vi "S4GUI_002.vi"(7 "Tab ObsEng":enum32{"Obs", "CCD modes", "Eng"}(tab)) -> ()   [LabVIEW 2018] (continued)
                n2402 = call "Next State.vi"("error in (no error)"=w4895, "New_State"=96, "State Machine in"=w4896) -> ("error out"=w4897:errorcluster, "State Machine out"=w4899:refnum<class "State Machine.lvclass">)  [unwired: 7 in]
                n2403 = call-dynamic "Write State Machine.vi"("error in (no error)"=w4897, "State Machine.lvclass"=w4899, "Device in"=w4900) -> ("error out"=w4902:errorcluster, "Device out"=w4903:refnum<class "Channel.lvclass">)  [unwired: 7 in]
                n2404 = call-dynamic "Write Channel.vi"("error in (no error)"=w4902, "Channel.lvclass"=w4903, "Acquisition in"=w4905) -> ("error out"=w4901:errorcluster, "Acquisition out"=w4904:refnum<class "Acquisition.lvclass">)  [unwired: 7 in]
              }
            }
            n2405 = call-dynamic "Write AcquisitionD.vi"("error in (no error)"=w4833, "Acquisition.lvclass"=w4834, "S4ACS_GUI in"=w4837) -> ("error out"=w4877:errorcluster, "S4ACS_GUI out"=w4878:refnum<class "S4GUI.lvclass">)  [unwired: 7 in]
          }
          frame True {
            # "vide S4GUI:\nHandleObservationSync.vi"
            # "aba atual em Tab Acq Type"
            n2406 = call "Read Instrument.lvclass.vi"("error in (no error)"=w4961, "S4ACS_GUI in"=w4962) -> ("error out"=w4964:errorcluster, "Instrument.lvclass"=w4966:refnum<class "Instrument.lvclass">, "S4ACS_GUI out"=w4959:refnum<class "S4GUI.lvclass">)  [unwired: 7 in]
            n2407 = call "Read WPROT.vi"("error in (no error)"=w4964, "Instrument in"=w4966) -> ("error out"=w4963:errorcluster, "Opt_Selector.lvclass"=w4965:refnum<class "Opt_Selector.lvclass">)  [unwired: 7 in, 1 out]
            n2408 = call-dynamic "Read sequencia.vi"("error in (no error)"=w4963, "Opt_Selector in"=w4965) -> ("error out"=w4958:errorcluster, "sequencia"=w4960:u16)  [unwired: 7 in, 1 out]
            n2409 = case shown="\"FOCUS\"" w4952 {
              tunnel: [u32 271 ("Obs_state") u32 251 ("Obs_state")] -> w4986
              tunnel: w4959 -> [w5007 w5010]
              tunnel: w4958 -> [w4997 w5009]
              tunnel: [w5005 w5010] -> w4957
              tunnel: [w4996 w5009] -> w4956
              tunnel: w4955 -> [w5004 _]
              tunnel: w4954 -> [w5003 _]
              tunnel: w4953 -> [w5002 _]
              frame "FOCUS" {
                n2410 = call-dynamic "Read TelFocus.lvclass.vi"("error in (no error)"=w4997, "S4GUI in"=w5007) -> ("error out"=w4999:errorcluster, "TelFocus.lvclass"=w5001:refnum<class "TelFocus.lvclass">, "S4GUI out"=w5006:refnum<class "S4GUI.lvclass">)  [unwired: 7 in]
                n2411 = call-dynamic "LoadParam.vi"("#steps"=w5002, "error in (no error)"=w4999, "step"=w5003, "init"=w5004, "TelFocus in"=w5001) -> ("error out"=w4998:errorcluster, "TelFocus out"=w5000:refnum<class "TelFocus.lvclass">)  [unwired: 5 in]
                n2412 = call-dynamic "Write TelFocus.lvclass.vi"("error in (no error)"=w4998, "TelFocus.lvclass"=w5000, "S4GUI in"=w5006) -> ("error out"=w4996:errorcluster, "S4GUI out"=w5005:refnum<class "S4GUI.lvclass">)  [unwired: 7 in]
              }
              frame Default {
              }
            }
            n2413 = case shown="Default" w4952 {
              tunnel: w4977 -> [_ w4992]
              tunnel: [u32 1 ("# Cycles") w4991] -> w4972
              tunnel: [u32 1 w4990] -> w4967
              tunnel: w4960 -> [_ w4989]
              frame "FOCUS" {
                # "Aba FOCUS: Para a sequencia de foco, sempre  #Cycles=1 e #Seqs=1"
              }
              frame Default {
                n2414 = case shown="True" w4992 {
                  tunnel: [0 w4995] -> w4990
                  tunnel: w4989 -> [_ w4994]
                  frame False {
                    # "OV 20230424: \n#SEQ agora armazena as\nposições da lâmina utilizadas.\nNa fotometria, #SEQ=0"
                    # "fotometria:"
                  }
                  frame True {
                    # "OV 20230424: \n#SEQ agora armazena as\nposições da lâmina utilizadas.\nNa polarimetria, #SEQ=WPROT.sequencia"
                    # "polarimetria:"
                    n2415 = To Unsigned Long Integer(number=w4994) -> (unsigned 32bit integer=w4995:u32)
                  }
                }
                n2416 = local read "# Cycles"() -> (w4991:u32)
              }
            }
            n2417 = call-dynamic "Write Obs_state.vi"("error in (no error)"=w4956, "Obs_state"=w4986, "S4ACS_GUI in"=w4957) -> ("error out"=w4985:errorcluster, "S4ACS_GUI out"=w4984:refnum<class "S4GUI.lvclass">)  [unwired: 7 in]
            n2418 = stacked-sequence {
              seq-local: [w5040 _ _ _] -> [_ w5126 _ _]
              seq-local: [w5039 _ _ _] -> [_ w5125 _ _]
              seq-local: [_ w5124 _ _] -> [_ _ w5187 _]
              seq-local: [_ w5123 _ _] -> [_ _ w5186 _]
              seq-local: [_ _ w5185 _] -> [_ _ _ w5248]
              seq-local: [_ _ w5184 _] -> [_ _ _ w5247]
              tunnel: w4985 -> [w5058 _ _ _]
              tunnel: w4984 -> [w5057 _ _ _]
              tunnel: [_ _ _ w5246] -> w4969
              tunnel: [_ _ _ w5245] -> w4971
              tunnel: w4982 -> [w5038 w5122 w5183 w5244]
              tunnel: w4981 -> [w5037 w5121 w5159 w5220]
              tunnel: w4980 -> [w5036 w5097 w5158 w5219]
              tunnel: w4979 -> [w5035 w5096 w5157 w5218]
              tunnel: w4978 -> [w5030 w5091 w5152 w5213]
              tunnel: w4972 -> [w5027 w5088 w5149 w5210]
              tunnel: w4967 -> [w5022 w5083 w5144 w5205]
              tunnel: w4952 -> [w5016 w5079 w5140 w5199]
              frame #0 {
                # "object"
                # "suffix"
                # "obsType"
                n2419 = local read "Exptime ch1"() -> (w5017:dbl)
                n2420 = call-dynamic "Read AcquisitionA.vi"("error in (no error)"=w5058, "S4ACS_GUI in"=w5057) -> ("error out"=w5056:errorcluster, "Acquisition.lvclass"=w5055:refnum<class "Acquisition.lvclass">, "S4ACS_GUI out"=w5045:refnum<class "S4GUI.lvclass">)  [unwired: 7 in]
                n2421 = call-dynamic "Read Channel.vi"("error in (no error)"=w5056, "Acquisition in"=w5055) -> ("error out"=w5053:errorcluster, "Channel.lvclass"=w5054:refnum<class "Channel.lvclass">, "Acquisition out"=w5044:refnum<class "Acquisition.lvclass">)  [unwired: 7 in]
                n2422 = local read "Exp ch1"() -> (w5042:u32)
                n2423 = call-dynamic "Read Interface.vi"("error in (no error)"=w5053, "Channel in"=w5054) -> ("error out"=w5065:errorcluster, "Interface.lvclass"=w5051:refnum<class "Interface.lvclass">, "Channel out"=w5052:refnum<class "Channel.lvclass">)  [unwired: 7 in]
                n2424 = call "Write Exposure Time.vi"("error in (no error)"=w5065, "Exposure Time"=w5017, "Interface in"=w5051) -> ("error out"=w5018:errorcluster, "Interface out"=w5021:refnum<class "Interface.lvclass">)  [unwired: 7 in]
                n2425 = case shown="Default" w5016 {
                  tunnel: w5021 -> [w5067 w5072]
                  tunnel: [w5067 w5071] -> w5020
                  tunnel: [w5066 w5070] -> w5019
                  tunnel: w5018 -> [w5066 w5069]
                  tunnel: w5017 -> [_ w5068]
                  frame "ZERO" {
                  }
                  frame Default {
                    n2426 = call-dynamic "Write prev ExpTime.vi"("error in (no error)"=w5069, "prev ExpTime"=w5068, "Interface in"=w5072) -> ("error out"=w5070:errorcluster, "Interface out"=w5071:refnum<class "Interface.lvclass">)  [unwired: 7 in]
                  }
                }
                n2427 = call-dynamic "Write Suffix.vi"("error in (no error)"=w5019, "Suffix"=w5038, "Interface in"=w5020) -> ("error out"=w5064:errorcluster, "Interface out"=w5050:refnum<class "Interface.lvclass">)  [unwired: 7 in]
                n2428 = call-dynamic "Write ObsType.vi"("error in (no error)"=w5064, "ObsType"=w5036, "Interface in"=w5050) -> ("error out"=w5063:errorcluster, "Interface out"=w5049:refnum<class "Interface.lvclass">)  [unwired: 7 in]
                n2429 = call-dynamic "Write Object.vi"("error in (no error)"=w5063, "Object"=w5035, "Interface in"=w5049) -> ("error out"=w5062:errorcluster, "Interface out"=w5048:refnum<class "Interface.lvclass">)  [unwired: 7 in]
                n2430 = call-dynamic "Write Comments.vi"("error in (no error)"=w5062, "Comments"=w5037, "Interface in"=w5048) -> ("error out"=w5061:errorcluster, "Interface out"=w5047:refnum<class "Interface.lvclass">)  [unwired: 7 in]
                n2431 = call-dynamic "Write DS9.vi"("error in (no error)"=w5061, "DS9"="F", "Interface in"=w5047) -> ("error out"=w5032:errorcluster, "Interface out"=w5034:refnum<class "Interface.lvclass">)  [unwired: 7 in]
                n2432 = call-dynamic "Write Observer.vi"("error in (no error)"=w5032, "Observer"=w5030, "Interface in"=w5034) -> ("error out"=w5031:errorcluster, "Interface out"=w5033:refnum<class "Interface.lvclass">)  [unwired: 7 in]
                n2433 = call-dynamic "Write # Images.vi"("error in (no error)"=w5031, "# Images"=w5042, "Interface in"=w5033) -> ("error out"=w5059:errorcluster, "Interface out"=w5046:refnum<class "Interface.lvclass">)  [unwired: 7 in]
                n2434 = property on="Exposures Done ch1" class="Slide (strict)"("Scale.Maximum"=w5042, "Scale.Minimum"=0.0 ("Scale.Range:Minimum")) -> ()  [unwired: 2 in, 2 out]
                n2435 = property on="Exposure Time ch1" class="Slide (strict)"("Scale.Maximum"=w5017, "Scale.Minimum"=0.0 ("Scale.Range:Minimum")) -> ()  [unwired: 2 in, 2 out]
                n2436 = call-dynamic "Write Interface.vi"("error in (no error)"=w5059, "Interface.lvclass"=w5046, "Channel in"=w5052) -> ("error out"=w5029:errorcluster, "Channel out"=w5028:refnum<class "Channel.lvclass">)  [unwired: 7 in]
                n2437 = call-dynamic "Write ciclos.vi"("error in (no error)"=w5029, "ciclos"=w5027, "Channel in"=w5028) -> ("error out"=w5024:errorcluster, "Channel out"=w5026:refnum<class "Channel.lvclass">)  [unwired: 7 in]
                n2438 = call-dynamic "Write sequencias.vi"("error in (no error)"=w5024, "sequencias"=w5022, "Channel in"=w5026) -> ("error out"=w5023:errorcluster, "Channel out"=w5025:refnum<class "Channel.lvclass">)  [unwired: 7 in]
                n2439 = call-dynamic "Write Channel.vi"("error in (no error)"=w5023, "Channel.lvclass"=w5025, "Acquisition in"=w5044) -> ("error out"=w5013:errorcluster, "Acquisition out"=w5015:refnum<class "Acquisition.lvclass">)  [unwired: 7 in]
                n2440 = call-dynamic "CalcCubeDuration.vi"("error in (no error)"=w5013, "Acquisition in"=w5015) -> ("error out"=w5012:errorcluster, "Acquisition out"=w5014:refnum<class "Acquisition.lvclass">)  [unwired: 8 in]
                n2441 = call-dynamic "Write AcquisitionA.vi"("error in (no error)"=w5012, "Acquisition.lvclass"=w5014, "S4ACS_GUI in"=w5045) -> ("error out"=w5039:errorcluster, "S4ACS_GUI out"=w5040:refnum<class "S4GUI.lvclass">)  [unwired: 7 in]
              }
              frame #1 {
                # "object"
                # "suffix"
                # "obsType"
                n2442 = call "Read AcquisitionB.vi"("error in (no error)"=w5125, "S4ACS_GUI in"=w5126) -> ("error out"=w5108:errorcluster, "Acquisition.lvclass"=w5109:refnum<class "Acquisition.lvclass">, "S4ACS_GUI out"=w5119:refnum<class "S4GUI.lvclass">)  [unwired: 7 in]
                n2443 = local read "Exptime ch2"() -> (w5080:dbl)
                n2444 = call-dynamic "Read Channel.vi"("error in (no error)"=w5108, "Acquisition in"=w5109) -> ("error out"=w5111:errorcluster, "Channel.lvclass"=w5110:refnum<class "Channel.lvclass">, "Acquisition out"=w5120:refnum<class "Acquisition.lvclass">)  [unwired: 7 in]
                n2445 = call-dynamic "Read Interface.vi"("error in (no error)"=w5111, "Channel in"=w5110) -> ("error out"=w5102:errorcluster, "Interface.lvclass"=w5113:refnum<class "Interface.lvclass">, "Channel out"=w5112:refnum<class "Channel.lvclass">)  [unwired: 7 in]
                n2446 = call "Write Exposure Time.vi"("error in (no error)"=w5102, "Exposure Time"=w5080, "Interface in"=w5113) -> ("error out"=w5081:errorcluster, "Interface out"=w5082:refnum<class "Interface.lvclass">)  [unwired: 7 in]
                n2447 = case shown="Default" w5079 {
                  tunnel: w5082 -> [w5128 w5133]
                  tunnel: [w5128 w5132] -> w5078
                  tunnel: [w5127 w5131] -> w5077
                  tunnel: w5081 -> [w5127 w5130]
                  tunnel: w5080 -> [_ w5129]
                  frame "ZERO" {
                  }
                  frame Default {
                    n2448 = call-dynamic "Write prev ExpTime.vi"("error in (no error)"=w5130, "prev ExpTime"=w5129, "Interface in"=w5133) -> ("error out"=w5131:errorcluster, "Interface out"=w5132:refnum<class "Interface.lvclass">)  [unwired: 7 in]
                  }
                }
                n2449 = call-dynamic "Write Suffix.vi"("error in (no error)"=w5077, "Suffix"=w5122, "Interface in"=w5078) -> ("error out"=w5103:errorcluster, "Interface out"=w5114:refnum<class "Interface.lvclass">)  [unwired: 7 in]
                n2450 = call-dynamic "Write ObsType.vi"("error in (no error)"=w5103, "ObsType"=w5097, "Interface in"=w5114) -> ("error out"=w5104:errorcluster, "Interface out"=w5115:refnum<class "Interface.lvclass">)  [unwired: 7 in]
                n2451 = call-dynamic "Write Object.vi"("error in (no error)"=w5104, "Object"=w5096, "Interface in"=w5115) -> ("error out"=w5105:errorcluster, "Interface out"=w5116:refnum<class "Interface.lvclass">)  [unwired: 7 in]
                n2452 = call-dynamic "Write Comments.vi"("error in (no error)"=w5105, "Comments"=w5121, "Interface in"=w5116) -> ("error out"=w5106:errorcluster, "Interface out"=w5117:refnum<class "Interface.lvclass">)  [unwired: 7 in]
                n2453 = local read "Exp ch2"() -> (w5100:u32)
                n2454 = call-dynamic "Write DS9.vi"("error in (no error)"=w5106, "DS9"="F", "Interface in"=w5117) -> ("error out"=w5093:errorcluster, "Interface out"=w5095:refnum<class "Interface.lvclass">)  [unwired: 7 in]
                n2455 = call-dynamic "Write Observer.vi"("error in (no error)"=w5093, "Observer"=w5091, "Interface in"=w5095) -> ("error out"=w5092:errorcluster, "Interface out"=w5094:refnum<class "Interface.lvclass">)  [unwired: 7 in]
                n2456 = call-dynamic "Write # Images.vi"("error in (no error)"=w5092, "# Images"=w5100, "Interface in"=w5094) -> ("error out"=w5107:errorcluster, "Interface out"=w5118:refnum<class "Interface.lvclass">)  [unwired: 7 in]
                n2457 = property on="Exposure Time ch2" class="Slide (strict)"("Scale.Maximum"=w5080, "Scale.Minimum"=0.0 ("Scale.Range:Minimum")) -> ()  [unwired: 2 in, 2 out]
                n2458 = property on="Exposures Done ch2" class="Slide (strict)"("Scale.Maximum"=w5100, "Scale.Minimum"=0.0 ("Scale.Range:Minimum")) -> ()  [unwired: 2 in, 2 out]
                n2459 = call-dynamic "Write Interface.vi"("error in (no error)"=w5107, "Interface.lvclass"=w5118, "Channel in"=w5112) -> ("error out"=w5090:errorcluster, "Channel out"=w5089:refnum<class "Channel.lvclass">)  [unwired: 7 in]
                n2460 = call-dynamic "Write ciclos.vi"("error in (no error)"=w5090, "ciclos"=w5088, "Channel in"=w5089) -> ("error out"=w5085:errorcluster, "Channel out"=w5087:refnum<class "Channel.lvclass">)  [unwired: 7 in]
                n2461 = call-dynamic "Write sequencias.vi"("error in (no error)"=w5085, "sequencias"=w5083, "Channel in"=w5087) -> ("error out"=w5084:errorcluster, "Channel out"=w5086:refnum<class "Channel.lvclass">)  [unwired: 7 in]
                n2462 = call-dynamic "Write Channel.vi"("error in (no error)"=w5084, "Channel.lvclass"=w5086, "Acquisition in"=w5120) -> ("error out"=w5074:errorcluster, "Acquisition out"=w5076:refnum<class "Acquisition.lvclass">)  [unwired: 7 in]
                n2463 = call-dynamic "CalcCubeDuration.vi"("error in (no error)"=w5074, "Acquisition in"=w5076) -> ("error out"=w5073:errorcluster, "Acquisition out"=w5075:refnum<class "Acquisition.lvclass">)  [unwired: 8 in]
                n2464 = call "Write AcquisitionB.vi"("error in (no error)"=w5073, "Acquisition.lvclass"=w5075, "S4ACS_GUI in"=w5119) -> ("error out"=w5123:errorcluster, "S4ACS_GUI out"=w5124:refnum<class "S4GUI.lvclass">)  [unwired: 7 in]
              }
              frame #2 {
                # "object"
                # "suffix"
                # "obsType"
                n2465 = call-dynamic "Read AcquisitionC.vi"("error in (no error)"=w5186, "S4ACS_GUI in"=w5187) -> ("error out"=w5176:errorcluster, "Acquisition.lvclass"=w5175:refnum<class "Acquisition.lvclass">, "S4ACS_GUI out"=w5165:refnum<class "S4GUI.lvclass">)  [unwired: 7 in]
                n2466 = call-dynamic "Read Channel.vi"("error in (no error)"=w5176, "Acquisition in"=w5175) -> ("error out"=w5173:errorcluster, "Channel.lvclass"=w5174:refnum<class "Channel.lvclass">, "Acquisition out"=w5164:refnum<class "Acquisition.lvclass">)  [unwired: 7 in]
                n2467 = local read "Exptime ch3"() -> (w5141:dbl)
                n2468 = call-dynamic "Read Interface.vi"("error in (no error)"=w5173, "Channel in"=w5174) -> ("error out"=w5182:errorcluster, "Interface.lvclass"=w5171:refnum<class "Interface.lvclass">, "Channel out"=w5172:refnum<class "Channel.lvclass">)  [unwired: 7 in]
                n2469 = call "Write Exposure Time.vi"("error in (no error)"=w5182, "Exposure Time"=w5141, "Interface in"=w5171) -> ("error out"=w5142:errorcluster, "Interface out"=w5143:refnum<class "Interface.lvclass">)  [unwired: 7 in]
                n2470 = case shown="\"ZERO\"" w5140 {
                  tunnel: w5143 -> [w5189 w5194]
                  tunnel: [w5189 w5193] -> w5139
                  tunnel: [w5188 w5192] -> w5138
                  tunnel: w5142 -> [w5188 w5191]
                  tunnel: w5141 -> [_ w5190]
                  frame "ZERO" {
                  }
                  frame Default {
                    n2471 = call-dynamic "Write prev ExpTime.vi"("error in (no error)"=w5191, "prev ExpTime"=w5190, "Interface in"=w5194) -> ("error out"=w5192:errorcluster, "Interface out"=w5193:refnum<class "Interface.lvclass">)  [unwired: 7 in]
                  }
                }
                n2472 = call-dynamic "Write Suffix.vi"("error in (no error)"=w5138, "Suffix"=w5183, "Interface in"=w5139) -> ("error out"=w5181:errorcluster, "Interface out"=w5170:refnum<class "Interface.lvclass">)  [unwired: 7 in]
                n2473 = call-dynamic "Write ObsType.vi"("error in (no error)"=w5181, "ObsType"=w5158, "Interface in"=w5170) -> ("error out"=w5180:errorcluster, "Interface out"=w5169:refnum<class "Interface.lvclass">)  [unwired: 7 in]
                n2474 = call-dynamic "Write Object.vi"("error in (no error)"=w5180, "Object"=w5157, "Interface in"=w5169) -> ("error out"=w5179:errorcluster, "Interface out"=w5168:refnum<class "Interface.lvclass">)  [unwired: 7 in]
                n2475 = call-dynamic "Write Comments.vi"("error in (no error)"=w5179, "Comments"=w5159, "Interface in"=w5168) -> ("error out"=w5178:errorcluster, "Interface out"=w5167:refnum<class "Interface.lvclass">)  [unwired: 7 in]
                n2476 = call-dynamic "Write DS9.vi"("error in (no error)"=w5178, "DS9"="F", "Interface in"=w5167) -> ("error out"=w5154:errorcluster, "Interface out"=w5156:refnum<class "Interface.lvclass">)  [unwired: 7 in]
                n2477 = local read "Exp ch3"() -> (w5162:u32)
                n2478 = property on="Exposure Time ch3" class="Slide (strict)"("Scale.Maximum"=w5141, "Scale.Minimum"=0.0 ("Scale.Range:Minimum")) -> ()  [unwired: 2 in, 2 out]
                n2479 = call-dynamic "Write Observer.vi"("error in (no error)"=w5154, "Observer"=w5152, "Interface in"=w5156) -> ("error out"=w5153:errorcluster, "Interface out"=w5155:refnum<class "Interface.lvclass">)  [unwired: 7 in]
                n2480 = property on="Exposures Done ch3" class="Slide (strict)"("Scale.Maximum"=w5162, "Scale.Minimum"=0.0 ("Scale.Range:Minimum")) -> ()  [unwired: 2 in, 2 out]
                n2481 = call-dynamic "Write # Images.vi"("error in (no error)"=w5153, "# Images"=w5162, "Interface in"=w5155) -> ("error out"=w5177:errorcluster, "Interface out"=w5166:refnum<class "Interface.lvclass">)  [unwired: 7 in]
                n2482 = call-dynamic "Write Interface.vi"("error in (no error)"=w5177, "Interface.lvclass"=w5166, "Channel in"=w5172) -> ("error out"=w5151:errorcluster, "Channel out"=w5150:refnum<class "Channel.lvclass">)  [unwired: 7 in]
                n2483 = call-dynamic "Write ciclos.vi"("error in (no error)"=w5151, "ciclos"=w5149, "Channel in"=w5150) -> ("error out"=w5146:errorcluster, "Channel out"=w5148:refnum<class "Channel.lvclass">)  [unwired: 7 in]
                n2484 = call-dynamic "Write sequencias.vi"("error in (no error)"=w5146, "sequencias"=w5144, "Channel in"=w5148) -> ("error out"=w5145:errorcluster, "Channel out"=w5147:refnum<class "Channel.lvclass">)  [unwired: 7 in]
                n2485 = call-dynamic "Write Channel.vi"("error in (no error)"=w5145, "Channel.lvclass"=w5147, "Acquisition in"=w5164) -> ("error out"=w5135:errorcluster, "Acquisition out"=w5137:refnum<class "Acquisition.lvclass">)  [unwired: 7 in]
                n2486 = call-dynamic "CalcCubeDuration.vi"("error in (no error)"=w5135, "Acquisition in"=w5137) -> ("error out"=w5134:errorcluster, "Acquisition out"=w5136:refnum<class "Acquisition.lvclass">)  [unwired: 8 in]
                n2487 = call-dynamic "Write AcquisitionC.vi"("error in (no error)"=w5134, "Acquisition.lvclass"=w5136, "S4ACS_GUI in"=w5165) -> ("error out"=w5184:errorcluster, "S4ACS_GUI out"=w5185:refnum<class "S4GUI.lvclass">)  [unwired: 7 in]
              }
              frame #3 {
                # "object"
                # "suffix"
                # "obsType"
                n2488 = call-dynamic "Read AcquisitionD.vi"("error in (no error)"=w5247, "S4ACS_GUI in"=w5248) -> ("error out"=w5237:errorcluster, "Acquisition.lvclass"=w5236:refnum<class "Acquisition.lvclass">, "S4ACS_GUI out"=w5226:refnum<class "S4GUI.lvclass">)  [unwired: 7 in]
                n2489 = local read "Exptime ch4"() -> (w5200:dbl)
                n2490 = call-dynamic "Read Channel.vi"("error in (no error)"=w5237, "Acquisition in"=w5236) -> ("error out"=w5234:errorcluster, "Channel.lvclass"=w5235:refnum<class "Channel.lvclass">, "Acquisition out"=w5225:refnum<class "Acquisition.lvclass">)  [unwired: 7 in]
                n2491 = call-dynamic "Read Interface.vi"("error in (no error)"=w5234, "Channel in"=w5235) -> ("error out"=w5243:errorcluster, "Interface.lvclass"=w5232:refnum<class "Interface.lvclass">, "Channel out"=w5233:refnum<class "Channel.lvclass">)  [unwired: 7 in]
                n2492 = call "Write Exposure Time.vi"("error in (no error)"=w5243, "Exposure Time"=w5200, "Interface in"=w5232) -> ("error out"=w5202:errorcluster, "Interface out"=w5204:refnum<class "Interface.lvclass">)  [unwired: 7 in]
                n2493 = case shown="Default" w5199 {
                  tunnel: w5204 -> [w5250 w5255]
                  tunnel: [w5250 w5254] -> w5203
                  tunnel: [w5249 w5253] -> w5201
                  tunnel: w5202 -> [w5249 w5252]
                  tunnel: w5200 -> [_ w5251]
                  frame "ZERO" {
                  }
                  frame Default {
                    n2494 = call-dynamic "Write prev ExpTime.vi"("error in (no error)"=w5252, "prev ExpTime"=w5251, "Interface in"=w5255) -> ("error out"=w5253:errorcluster, "Interface out"=w5254:refnum<class "Interface.lvclass">)  [unwired: 7 in]
                  }
                }
                n2495 = call-dynamic "Write Suffix.vi"("error in (no error)"=w5201, "Suffix"=w5244, "Interface in"=w5203) -> ("error out"=w5242:errorcluster, "Interface out"=w5231:refnum<class "Interface.lvclass">)  [unwired: 7 in]
                n2496 = call-dynamic "Write ObsType.vi"("error in (no error)"=w5242, "ObsType"=w5219, "Interface in"=w5231) -> ("error out"=w5241:errorcluster, "Interface out"=w5230:refnum<class "Interface.lvclass">)  [unwired: 7 in]
                n2497 = call-dynamic "Write Object.vi"("error in (no error)"=w5241, "Object"=w5218, "Interface in"=w5230) -> ("error out"=w5240:errorcluster, "Interface out"=w5229:refnum<class "Interface.lvclass">)  [unwired: 7 in]
                n2498 = call-dynamic "Write Comments.vi"("error in (no error)"=w5240, "Comments"=w5220, "Interface in"=w5229) -> ("error out"=w5239:errorcluster, "Interface out"=w5228:refnum<class "Interface.lvclass">)  [unwired: 7 in]
                n2499 = call-dynamic "Write DS9.vi"("error in (no error)"=w5239, "DS9"="F", "Interface in"=w5228) -> ("error out"=w5215:errorcluster, "Interface out"=w5217:refnum<class "Interface.lvclass">)  [unwired: 7 in]
                n2500 = property on="Exposure Time ch4" class="Slide (strict)"("Scale.Maximum"=w5200, "Scale.Minimum"=0.0 ("Scale.Range:Minimum")) -> ()  [unwired: 2 in, 2 out]
                n2501 = local read "Exp ch4"() -> (w5223:u32)
                n2502 = call-dynamic "Write Observer.vi"("error in (no error)"=w5215, "Observer"=w5213, "Interface in"=w5217) -> ("error out"=w5214:errorcluster, "Interface out"=w5216:refnum<class "Interface.lvclass">)  [unwired: 7 in]
                n2503 = property on="Exposures Done ch4" class="Slide (strict)"("Scale.Maximum"=w5223, "Scale.Minimum"=0.0 ("Scale.Range:Minimum")) -> ()  [unwired: 2 in, 2 out]
                n2504 = call-dynamic "Write # Images.vi"("error in (no error)"=w5214, "# Images"=w5223, "Interface in"=w5216) -> ("error out"=w5238:errorcluster, "Interface out"=w5227:refnum<class "Interface.lvclass">)  [unwired: 7 in]
                n2505 = call-dynamic "Write Interface.vi"("error in (no error)"=w5238, "Interface.lvclass"=w5227, "Channel in"=w5233) -> ("error out"=w5212:errorcluster, "Channel out"=w5211:refnum<class "Channel.lvclass">)  [unwired: 7 in]
                n2506 = call-dynamic "Write ciclos.vi"("error in (no error)"=w5212, "ciclos"=w5210, "Channel in"=w5211) -> ("error out"=w5208:errorcluster, "Channel out"=w5209:refnum<class "Channel.lvclass">)  [unwired: 7 in]
                n2507 = call-dynamic "Write sequencias.vi"("error in (no error)"=w5208, "sequencias"=w5205, "Channel in"=w5209) -> ("error out"=w5207:errorcluster, "Channel out"=w5206:refnum<class "Channel.lvclass">)  [unwired: 7 in]
                n2508 = call-dynamic "Write Channel.vi"("error in (no error)"=w5207, "Channel.lvclass"=w5206, "Acquisition in"=w5225) -> ("error out"=w5196:errorcluster, "Acquisition out"=w5198:refnum<class "Acquisition.lvclass">)  [unwired: 7 in]
                n2509 = call-dynamic "CalcCubeDuration.vi"("error in (no error)"=w5196, "Acquisition in"=w5198) -> ("error out"=w5195:errorcluster, "Acquisition out"=w5197:refnum<class "Acquisition.lvclass">)  [unwired: 8 in]
                n2510 = call-dynamic "Write AcquisitionD.vi"("error in (no error)"=w5195, "Acquisition.lvclass"=w5197, "S4ACS_GUI in"=w5226) -> ("error out"=w5245:errorcluster, "S4ACS_GUI out"=w5246:refnum<class "S4GUI.lvclass">)  [unwired: 7 in]
              }
            }
            n2511 = call-dynamic "Write sequencias.vi"("error in (no error)"=w4971, "sequencias"=w4967, "S4GUI in"=w4969) -> ("error out"=w4970:errorcluster, "S4GUI out"=w4968:refnum<class "S4GUI.lvclass">)  [unwired: 7 in]
            n2512 = call-dynamic "Write ciclos.vi"("error in (no error)"=w4970, "ciclos"=w4972, "S4ACS_GUI in"=w4968) -> ("error out"=w4974:errorcluster, "S4ACS_GUI out"=w4976:refnum<class "S4GUI.lvclass">)  [unwired: 7 in]
            n2513 = property on="#Cycles Done" class="Slide (strict)"("Scale.Maximum"=w4972, "Scale.Minimum"=0.0 ("Scale.Range:Minor Increment")) -> ()  [unwired: 2 in, 2 out]
            n2514 = call-dynamic "Write TotalCiclos.vi"("error in (no error)"=w4974, "TotalCiclos"=w4972, "S4GUI in"=w4976) -> ("error out"=w4973:errorcluster, "S4GUI out"=w4975:refnum<class "S4GUI.lvclass">)  [unwired: 7 in]
          }
        }
        n2515 = call-dynamic "Write User Event.vi"("error in (no error)"=w4808, "User Event"=w4805, "S4GUI in"=w4809) -> ("error out"=w4807:errorcluster, "S4GUI out"=w4806:refnum<class "S4GUI.lvclass">)  [unwired: 7 in]
        n2516 = property on="Pause SM" class="Bool"(error in=w4807, "DisabledEnum"=T12."Enabled" ("Disabled")) -> (error out=w4826:errorcluster)  [unwired: 1 in, 1 out]
      }
      event "# Cycles": Value Change {
        w5256 = 0.0 ("Scale.Range:Minor Increment")
        n2517 = event-data() -> ("NewVal"=w5257:u32)  [unwired: 1 in]
        n2518 = call-dynamic "Write ciclos.vi"("error in (no error)"=w5260, "ciclos"=w5257, "S4ACS_GUI in"=w5261) -> ("error out"=w5259:errorcluster, "S4ACS_GUI out"=w5258:refnum<class "S4GUI.lvclass">)  [unwired: 7 in]
        n2519 = property on="#Cycles Done" class="Slide (strict)"("Scale.Maximum"=w5257, "Scale.Minimum"=w5256) -> ()  [unwired: 2 in, 2 out]
        n2520 = property on="Cycles Done ch2" class="Slide (strict)"("Scale.Maximum"=w5257, "Scale.Minimum"=w5256) -> ()  [unwired: 2 in, 2 out]
        n2521 = property on="Cycles Done ch4" class="Slide (strict)"("Scale.Maximum"=w5257, "Scale.Minimum"=w5256) -> ()  [unwired: 2 in, 2 out]
        n2522 = property on="Cycles Done ch1" class="Slide (strict)"("Scale.Maximum"=w5257, "Scale.Minimum"=w5256) -> ()  [unwired: 2 in, 2 out]
        n2523 = property on="Cycles Done ch3" class="Slide (strict)"("Scale.Maximum"=w5257, "Scale.Minimum"=w5256) -> ()  [unwired: 2 in, 2 out]
      }
      event "AllConfig": Value Change {
        n2524 = event-data() -> ()  [unwired: 1 in, 6 out]
        n2525 = call "Read Instrument.lvclass.vi"("error in (no error)"=w5266, "S4ACS_GUI in"=w5267) -> ("error out"=w5346:errorcluster, "Instrument.lvclass"=w5313:refnum<class "Instrument.lvclass">, "S4ACS_GUI out"=w5344:refnum<class "S4GUI.lvclass">)  [unwired: 7 in]
        n2526 = call "Read ASEL.vi"("error in (no error)"=w5346, "Instrument in"=w5313) -> ("error out"=w5338:errorcluster, "Opt_Selector.lvclass"=w5337:refnum<class "Opt_Selector.lvclass">, "Instrument out"=w5345:refnum<class "Instrument.lvclass">)  [unwired: 7 in]
        n2527 = call-dynamic "Read State Machine.vi"("error in (no error)"=w5338, "Device in"=w5337) -> ("error out"=w5341:errorcluster, "State Machine.lvclass"=w5343:refnum<class "State Machine.lvclass">, "Device out"=w5335:refnum<class "Opt_Selector.lvclass">)  [unwired: 7 in]
        n2528 = call "Next State.vi"("error in (no error)"=w5341, "New_State"=1, "State Machine in"=w5343) -> ("error out"=w5340:errorcluster, "State Machine out"=w5339:refnum<class "State Machine.lvclass">)  [unwired: 7 in]
        n2529 = call-dynamic "Write State Machine.vi"("error in (no error)"=w5340, "State Machine.lvclass"=w5339, "Device in"=w5335) -> ("error out"=w5334:errorcluster, "Device out"=w5336:refnum<class "Opt_Selector.lvclass">)  [unwired: 7 in]
        n2530 = call "Write ASEL.vi"("error in (no error)"=w5334, "Opt_Selector.lvclass"=w5336, "Instrument in"=w5345) -> ("error out"=w5296:errorcluster, "Instrument out"=w5312:refnum<class "Instrument.lvclass">)  [unwired: 7 in]
        n2531 = call "Read CALW.vi"("error in (no error)"=w5296, "Instrument in"=w5312) -> ("error out"=w5329:errorcluster, "Opt_Selector.lvclass"=w5330:refnum<class "Opt_Selector.lvclass">, "Instrument out"=w5311:refnum<class "Instrument.lvclass">)  [unwired: 7 in]
        n2532 = call-dynamic "Read State Machine.vi"("error in (no error)"=w5329, "Device in"=w5330) -> ("error out"=w5326:errorcluster, "State Machine.lvclass"=w5324:refnum<class "State Machine.lvclass">, "Device out"=w5332:refnum<class "Opt_Selector.lvclass">)  [unwired: 7 in]
        n2533 = call "Next State.vi"("error in (no error)"=w5326, "New_State"=1, "State Machine in"=w5324) -> ("error out"=w5327:errorcluster, "State Machine out"=w5328:refnum<class "State Machine.lvclass">)  [unwired: 7 in]
        n2534 = call-dynamic "Write State Machine.vi"("error in (no error)"=w5327, "State Machine.lvclass"=w5328, "Device in"=w5332) -> ("error out"=w5333:errorcluster, "Device out"=w5331:refnum<class "Opt_Selector.lvclass">)  [unwired: 7 in]
        n2535 = call "Write CALW.vi"("error in (no error)"=w5333, "Opt_Selector.lvclass"=w5331, "Instrument in"=w5311) -> ("error out"=w5295:errorcluster, "Instrument out"=w5310:refnum<class "Instrument.lvclass">)  [unwired: 7 in]
        n2536 = call "Read WPSEL.vi"("error in (no error)"=w5295, "Instrument in"=w5310) -> ("error out"=w5318:errorcluster, "Opt_Selector.lvclass"=w5317:refnum<class "Opt_Selector.lvclass">, "Instrument out"=w5309:refnum<class "Instrument.lvclass">)  [unwired: 7 in]
        n2537 = call-dynamic "Read State Machine.vi"("error in (no error)"=w5318, "Device in"=w5317) -> ("error out"=w5321:errorcluster, "State Machine.lvclass"=w5323:refnum<class "State Machine.lvclass">, "Device out"=w5315:refnum<class "Opt_Selector.lvclass">)  [unwired: 7 in]
        n2538 = call "Next State.vi"("error in (no error)"=w5321, "New_State"=1, "State Machine in"=w5323) -> ("error out"=w5320:errorcluster, "State Machine out"=w5319:refnum<class "State Machine.lvclass">)  [unwired: 7 in]
        n2539 = call-dynamic "Write State Machine.vi"("error in (no error)"=w5320, "State Machine.lvclass"=w5319, "Device in"=w5315) -> ("error out"=w5314:errorcluster, "Device out"=w5316:refnum<class "Opt_Selector.lvclass">)  [unwired: 7 in]
        n2540 = call "Write WPSEL.vi"("error in (no error)"=w5314, "Opt_Selector.lvclass"=w5316, "Instrument in"=w5309) -> ("error out"=w5294:errorcluster, "Instrument out"=w5298:refnum<class "Instrument.lvclass">)  [unwired: 7 in]
        n2541 = call "Read WPROT.vi"("error in (no error)"=w5294, "Instrument in"=w5298) -> ("error out"=w5304:errorcluster, "Opt_Selector.lvclass"=w5305:refnum<class "Opt_Selector.lvclass">, "Instrument out"=w5297:refnum<class "Instrument.lvclass">)  [unwired: 7 in]
        n2542 = call-dynamic "Read State Machine.vi"("error in (no error)"=w5304, "Device in"=w5305) -> ("error out"=w5301:errorcluster, "State Machine.lvclass"=w5299:refnum<class "State Machine.lvclass">, "Device out"=w5307:refnum<class "Opt_Selector.lvclass">)  [unwired: 7 in]
        n2543 = call "Next State.vi"("error in (no error)"=w5301, "New_State"=1, "State Machine in"=w5299) -> ("error out"=w5302:errorcluster, "State Machine out"=w5303:refnum<class "State Machine.lvclass">)  [unwired: 7 in]
        n2544 = call-dynamic "Write State Machine.vi"("error in (no error)"=w5302, "State Machine.lvclass"=w5303, "Device in"=w5307) -> ("error out"=w5308:errorcluster, "Device out"=w5306:refnum<class "Opt_Selector.lvclass">)  [unwired: 7 in]
        n2545 = call "Write WPROT.vi"("error in (no error)"=w5308, "Opt_Selector.lvclass"=w5306, "Instrument in"=w5297) -> ("error out"=w5270:errorcluster, "Instrument out"=w5271:refnum<class "Instrument.lvclass">)  [unwired: 7 in]
        n2546 = call "Read GMIR.vi"("error in (no error)"=w5270, "Instrument in"=w5271) -> ("error out"=w5289:errorcluster, "Opt_Continuous.lvclass"=w5290:refnum<class "Opt_Continuous.lvclass">, "Instrument out"=w5283:refnum<class "Instrument.lvclass">)  [unwired: 7 in]
        n2547 = call-dynamic "Read State Machine.vi"("error in (no error)"=w5289, "Device in"=w5290) -> ("error out"=w5286:errorcluster, "State Machine.lvclass"=w5284:refnum<class "State Machine.lvclass">, "Device out"=w5292:refnum<class "Opt_Continuous.lvclass">)  [unwired: 7 in]
        n2548 = call "Next State.vi"("error in (no error)"=w5286, "New_State"=1, "State Machine in"=w5284) -> ("error out"=w5287:errorcluster, "State Machine out"=w5288:refnum<class "State Machine.lvclass">)  [unwired: 7 in]
        n2549 = call-dynamic "Write State Machine.vi"("error in (no error)"=w5287, "State Machine.lvclass"=w5288, "Device in"=w5292) -> ("error out"=w5293:errorcluster, "Device out"=w5291:refnum<class "Opt_Continuous.lvclass">)  [unwired: 7 in]
        n2550 = call "Write GMIR.vi"("error in (no error)"=w5293, "Opt_Continuous.lvclass"=w5291, "Instrument in"=w5283) -> ("error out"=w5268:errorcluster, "Instrument out"=w5269:refnum<class "Instrument.lvclass">)  [unwired: 7 in]
        n2551 = call "Read GFOC.vi"("error in (no error)"=w5268, "Instrument in"=w5269) -> ("error out"=w5278:errorcluster, "Opt_Continuous.lvclass"=w5279:refnum<class "Opt_Continuous.lvclass">, "Instrument out"=w5272:refnum<class "Instrument.lvclass">)  [unwired: 7 in]
        n2552 = call-dynamic "Read State Machine.vi"("error in (no error)"=w5278, "Device in"=w5279) -> ("error out"=w5275:errorcluster, "State Machine.lvclass"=w5273:refnum<class "State Machine.lvclass">, "Device out"=w5281:refnum<class "Opt_Continuous.lvclass">)  [unwired: 7 in]
        n2553 = call "Next State.vi"("error in (no error)"=w5275, "New_State"=1, "State Machine in"=w5273) -> ("error out"=w5276:errorcluster, "State Machine out"=w5277:refnum<class "State Machine.lvclass">)  [unwired: 7 in]
        n2554 = call-dynamic "Write State Machine.vi"("error in (no error)"=w5276, "State Machine.lvclass"=w5277, "Device in"=w5281) -> ("error out"=w5282:errorcluster, "Device out"=w5280:refnum<class "Opt_Continuous.lvclass">)  [unwired: 7 in]
        n2555 = call "Write GFOC.vi"("error in (no error)"=w5282, "Opt_Continuous.lvclass"=w5280, "Instrument in"=w5272) -> ("error out"=w5264:errorcluster, "Instrument out"=w5265:refnum<class "Instrument.lvclass">)  [unwired: 7 in]
        n2556 = call "Write Instrument.lvclass.vi"("error in (no error)"=w5264, "Instrument.lvclass"=w5265, "S4ACS_GUI in"=w5344) -> ("error out"=w5263:errorcluster, "S4ACS_GUI out"=w5262:refnum<class "S4GUI.lvclass">)  [unwired: 7 in]
      }
      event "Tab Acq Type": Value Change {
        # "Tab for choosing EXPOSURE MODE: Object, Dflat, Sflat, Dark, Zero, Focus"
        n2557 = event-data() -> ("NewVal"=w5385:T1)  [unwired: 1 in]
        n2558 = local read "Observer"() -> (w5383:string)
        n2559 = case shown="\"DFLAT\"" w5385 {
          tunnel: ["OBJECT" "FLAT" "FLAT" "DARK" "ZERO" "FOCUS"] -> w5362
          tunnel: [w5457 w5462 w5467 w5472 w5477 w5482] -> w5361
          tunnel: [w5456 w5461 w5466 w5471 w5476 w5481] -> w5384
          tunnel: [w5455 w5460 w5465 w5470 w5475 w5480] -> w5358
          tunnel: [u32 0 u32 1 u32 2 u32 3 u32 4 u32 5] -> w5353
          frame "OBJECT", Default {
            n2560 = local read "Object_obj"() -> (w5457:string)
            n2561 = local read "OBJECT Comments"() -> (w5455:string)
            n2562 = local read "object suffix"() -> (w5456:string)
          }
          frame "DFLAT" {
            n2563 = local read "DFLAT Comments"() -> (w5460:string)
            n2564 = local read "Object_dflat"() -> (w5462:string)
            n2565 = local read "dflat suffix"() -> (w5461:string)
          }
          frame "SFLAT" {
            n2566 = local read "SFLAT Comments"() -> (w5465:string)
            n2567 = local read "Object_sflat"() -> (w5467:string)
            n2568 = local read "sflat suffix"() -> (w5466:string)
          }
          frame "DARK" {
            n2569 = local read "Object_dark"() -> (w5472:string)
            n2570 = local read "dark suffix"() -> (w5471:string)
            n2571 = local read "DARK Comments"() -> (w5470:string)
          }
          frame "ZERO" {
            n2572 = local read "ZERO Comments"() -> (w5475:string)
            n2573 = local read "Object_zero"() -> (w5477:string)
            n2574 = local read "zero suffix"() -> (w5476:string)
          }
          frame "FOCUS" {
            n2575 = local read "FOCUS Comments"() -> (w5480:string)
            n2576 = local read "Object_focus"() -> (w5482:string)
            n2577 = local read "focus suffix"() -> (w5481:string)
          }
        }
        n2578 = call-dynamic "Write ExpMode.vi"("error in (no error)"=w5386, "ExpMode"=w5385, "S4GUI in"=w5387) -> ("error out"=w5379:errorcluster, "S4GUI out"=w5378:refnum<class "S4GUI.lvclass">)  [unwired: 7 in]
        n2579 = Concatenate Strings("ACQ TAB SELECTED:" ("User Event"), w5362) -> (w5380:string)
        n2580 = call-dynamic "Write User Event.vi"("error in (no error)"=w5379, "User Event"=w5380, "S4GUI in"=w5378) -> ("error out"=w5352:errorcluster, "S4GUI out"=w5351:refnum<class "S4GUI.lvclass">)  [unwired: 7 in]
        n2581 = call-dynamic "Write TabAcqType index.vi"("error in (no error)"=w5352, "TabAcqType index"=w5353, "S4GUI in"=w5351) -> ("error out"=w5348:errorcluster, "S4GUI out"=w5350:refnum<class "S4GUI.lvclass">)  [unwired: 7 in]
        n2582 = call-dynamic "Save TabAcqType index.vi"("error in (no error)"=w5348, "S4GUI in"=w5350) -> ("error out"=w5347:errorcluster, "S4GUI out"=w5349:refnum<class "S4GUI.lvclass">)  [unwired: 8 in]
        n2583 = call-dynamic "Read Publisher.lvclass.vi"("error in (no error)"=w5347, "S4GUI in"=w5349) -> ("error out"=w5376:errorcluster, "Publisher.lvclass"=w5372:refnum<class "Publisher.lvclass">, "S4GUI out"=w5377:refnum<class "S4GUI.lvclass">)  [unwired: 7 in]
        n2584 = call-dynamic "Write object.vi"("error in (no error)"=w5376, "object"=w5361, "Publisher in"=w5372) -> ("error out"=w5375:errorcluster, "Publisher out"=w5371:refnum<class "Publisher.lvclass">)  [unwired: 7 in]
        n2585 = call-dynamic "Write obstype.vi"("error in (no error)"=w5375, "obstype"=w5362, "Publisher in"=w5371) -> ("error out"=w5374:errorcluster, "Publisher out"=w5370:refnum<class "Publisher.lvclass">)  [unwired: 7 in]
        n2586 = call-dynamic "Write observer.vi"("error in (no error)"=w5374, "observer"=w5360, "Publisher in"=w5370) -> ("error out"=w5373:errorcluster, "Publisher out"=w5369:refnum<class "Publisher.lvclass">)  [unwired: 7 in]
        n2587 = call-dynamic "Write projid.vi"("error in (no error)"=w5373, "projid"=w5359, "Publisher in"=w5369) -> ("error out"=w5366:errorcluster, "Publisher out"=w5365:refnum<class "Publisher.lvclass">)  [unwired: 7 in]
        n2588 = call-dynamic "Write comments.vi"("error in (no error)"=w5366, "comments"=w5358, "Publisher in"=w5365) -> ("error out"=w5368:errorcluster, "Publisher out"=w5367:refnum<class "Publisher.lvclass">)  [unwired: 7 in]
        n2589 = call-dynamic "Write Publisher.lvclass.vi"("error in (no error)"=w5368, "Publisher.lvclass"=w5367, "S4GUI in"=w5377) -> ("error out"=w5364:errorcluster, "S4GUI out"=w5363:refnum<class "S4GUI.lvclass">)  [unwired: 7 in]
        n2590 = call-dynamic "Read AcquisitionA.vi"("error in (no error)"=w5364, "S4ACS_GUI in"=w5363) -> ("error out"=w5394:errorcluster, "Acquisition.lvclass"=w5395:refnum<class "Acquisition.lvclass">, "S4ACS_GUI out"=w5414:refnum<class "S4GUI.lvclass">)  [unwired: 7 in]
        n2591 = call-dynamic "Read AcquisitionC.vi"("error in (no error)"=w5352, "S4ACS_GUI in"=w5351) -> ("error out"=w5390:errorcluster, "Acquisition.lvclass"=w5391:refnum<class "Acquisition.lvclass">)  [unwired: 7 in, 1 out]
        n2592 = call "Read AcquisitionB.vi"("error in (no error)"=w5352, "S4ACS_GUI in"=w5351) -> ("error out"=w5392:errorcluster, "Acquisition.lvclass"=w5393:refnum<class "Acquisition.lvclass">)  [unwired: 7 in, 1 out]
        n2593 = call-dynamic "Read AcquisitionD.vi"("error in (no error)"=w5352, "S4ACS_GUI in"=w5351) -> ("error out"=w5388:errorcluster, "Acquisition.lvclass"=w5389:refnum<class "Acquisition.lvclass">)  [unwired: 7 in, 1 out]
        n2594 = To Lower Case(string=w5384) -> (all lower case string=w5382:string)
        n2595 = case shown="\"DARK\"" w5385 {
          tunnel: [w5717 w6086 w6471] -> w5413
          tunnel: [w5716 w6085 w6470] -> w5412
          tunnel: [w5715 w6084 w6469] -> w5410
          tunnel: [w5714 w6083 w6468] -> w5409
          tunnel: [w5713 w6082 w6467] -> w5399
          tunnel: [w5712 w6081 w6466] -> w5398
          tunnel: [w5711 w6080 w6465] -> w5397
          tunnel: [w5710 w6079 w6464] -> w5396
          tunnel: w5395 -> [w5709 w6078 w6463]
          tunnel: w5394 -> [w5708 w6077 w6462]
          tunnel: w5393 -> [w5698 w6068 w6453]
          tunnel: w5392 -> [w5697 w6067 w6452]
          tunnel: w5391 -> [w5696 w6066 w6451]
          tunnel: w5390 -> [w5695 w6065 w6450]
          tunnel: w5389 -> [w5694 w6064 w6449]
          tunnel: w5388 -> [w5693 w6063 w6448]
          tunnel: w5361 -> [w5690 w6062 w6447]
          tunnel: w5358 -> [w5691 w6061 w6446]
          tunnel: w5383 -> [w5692 w6060 w6445]
          tunnel: w5382 -> [w5689 w6059 w6444]
          tunnel: w5362 -> [w5688 w6058 w6443]
          frame "ZERO" {
            w5707 = 1e-05 ("Exptime ch1")
            # "nome do arquivo .cfg"
            # "seção no arquivo .cfg"
            # "nome do arquivo .cfg"
            # "seção no arquivo .cfg"
            # "nome do arquivo .cfg"
            # "seção no arquivo .cfg"
            # "nome do arquivo .cfg"
            # "seção no arquivo .cfg"
            # "ZERO: EXPTIME=1E-5 (mandatory), shutter automatically closed, save current FRAME_TRANSFER (prev_FT) and reset FRAME_TRANSFER."
            n2596 = call "Read connection.vi"("error in (no error)"=w5695, "Server in"=w5696) -> ("error out"=w5701:errorcluster, "connection"=w5535:bool, "Server out"=w5702:refnum<class "Acquisition.lvclass">)  [unwired: 7 in]
            n2597 = call "Read connection.vi"("error in (no error)"=w5697, "Server in"=w5698) -> ("error out"=w5703:errorcluster, "connection"=w5586:bool, "Server out"=w5704:refnum<class "Acquisition.lvclass">)  [unwired: 7 in]
            n2598 = call "Read connection.vi"("error in (no error)"=w5708, "Server in"=w5709) -> ("error out"=w5705:errorcluster, "connection"=w5637:bool, "Server out"=w5706:refnum<class "Acquisition.lvclass">)  [unwired: 7 in]
            n2599 = call "Read connection.vi"("error in (no error)"=w5693, "Server in"=w5694) -> ("error out"=w5699:errorcluster, "connection"=w5484:bool, "Server out"=w5700:refnum<class "Acquisition.lvclass">)  [unwired: 7 in]
            n2600 = call-dynamic "Read Channel.vi"("error in (no error)"=w5703, "Acquisition in"=w5704) -> ("error out"=w5624:errorcluster, "Channel.lvclass"=w5623:refnum<class "Channel.lvclass">, "Acquisition out"=w5622:refnum<class "Acquisition.lvclass">)  [unwired: 7 in]
            n2601 = call-dynamic "Read Channel.vi"("error in (no error)"=w5699, "Acquisition in"=w5700) -> ("error out"=w5532:errorcluster, "Channel.lvclass"=w5533:refnum<class "Channel.lvclass">, "Acquisition out"=w5534:refnum<class "Acquisition.lvclass">)  [unwired: 7 in]
            n2602 = call-dynamic "Read Channel.vi"("error in (no error)"=w5701, "Acquisition in"=w5702) -> ("error out"=w5573:errorcluster, "Channel.lvclass"=w5572:refnum<class "Channel.lvclass">, "Acquisition out"=w5571:refnum<class "Acquisition.lvclass">)  [unwired: 7 in]
            n2603 = call-dynamic "Read Channel.vi"("error in (no error)"=w5705, "Acquisition in"=w5706) -> ("error out"=w5685:errorcluster, "Channel.lvclass"=w5686:refnum<class "Channel.lvclass">, "Acquisition out"=w5687:refnum<class "Acquisition.lvclass">)  [unwired: 7 in]
            n2604 = call-dynamic "Read Interface.vi"("error in (no error)"=w5532, "Channel in"=w5533) -> ("error out"=w5498:errorcluster, "Interface.lvclass"=w5497:refnum<class "Interface.lvclass">, "Channel out"=w5494:refnum<class "Channel.lvclass">)  [unwired: 7 in]
            n2605 = call-dynamic "Read Interface.vi"("error in (no error)"=w5624, "Channel in"=w5623) -> ("error out"=w5598:errorcluster, "Interface.lvclass"=w5599:refnum<class "Interface.lvclass">, "Channel out"=w5593:refnum<class "Channel.lvclass">)  [unwired: 7 in]
            n2606 = call-dynamic "Read Interface.vi"("error in (no error)"=w5573, "Channel in"=w5572) -> ("error out"=w5547:errorcluster, "Interface.lvclass"=w5548:refnum<class "Interface.lvclass">, "Channel out"=w5545:refnum<class "Channel.lvclass">)  [unwired: 7 in]
            n2607 = call-dynamic "Read Interface.vi"("error in (no error)"=w5685, "Channel in"=w5686) -> ("error out"=w5654:errorcluster, "Interface.lvclass"=w5655:refnum<class "Interface.lvclass">, "Channel out"=w5648:refnum<class "Channel.lvclass">)  [unwired: 7 in]
            n2608 = call-dynamic "Write restoreExpTime.vi"("error in (no error)"=w5498, "restoreExpTime"=TRUE, "Interface in"=w5497) -> ("error out"=w5491:errorcluster, "Interface out"=w5496:refnum<class "Interface.lvclass">)  [unwired: 7 in]
            n2609 = property on="Exptime ch1" class="DigNum (strict)"("Value"=w5707) -> ()  [unwired: 2 in, 2 out]
            n2610 = call-dynamic "Write restoreExpTime.vi"("error in (no error)"=w5598, "restoreExpTime"=TRUE, "Interface in"=w5599) -> ("error out"=w5595:errorcluster, "Interface out"=w5597:refnum<class "Interface.lvclass">)  [unwired: 7 in]
            n2611 = call-dynamic "Write restoreExpTime.vi"("error in (no error)"=w5547, "restoreExpTime"=TRUE, "Interface in"=w5548) -> ("error out"=w5540:errorcluster, "Interface out"=w5546:refnum<class "Interface.lvclass">)  [unwired: 7 in]
            n2612 = call-dynamic "Write restoreExpTime.vi"("error in (no error)"=w5654, "restoreExpTime"=TRUE, "Interface in"=w5655) -> ("error out"=w5644:errorcluster, "Interface out"=w5645:refnum<class "Interface.lvclass">)  [unwired: 7 in]
            n2613 = call-dynamic "Read target cluster.vi"("error in (no error)"=w5595, "Channel in"=w5593) -> ("error out"=w5594:errorcluster, "target cluster"=w5596:T31, "Channel out"=w5589:refnum<class "Channel.lvclass">)  [unwired: 7 in]
            n2614 = stacked-sequence {
              tunnel: [_ w5809] -> w5592
              tunnel: w5596 -> [_ w5808]
              tunnel: w5596 -> [w5806 _]
              tunnel: [w5805 _] -> w5601
              frame #0 {
                n2615 = Unbundle By Name(w5806) -> ("FRAME_TRANSFER"=w5805:bool)
              }
              frame #1 {
                # "closed"
                n2616 = Bundle By Name(cluster=w5808, "SHUTTER_MODE"=u8 2, "FRAME_TRANSFER"=FALSE) -> (w5809:T31)
              }
            }
            n2617 = call-dynamic "Read target cluster.vi"("error in (no error)"=w5491, "Channel in"=w5494) -> ("error out"=w5490:errorcluster, "target cluster"=w5492:T31, "Channel out"=w5493:refnum<class "Channel.lvclass">)  [unwired: 7 in]
            n2618 = stacked-sequence {
              tunnel: w5492 -> [_ w5748]
              tunnel: [_ w5747] -> w5488
              tunnel: w5492 -> [w5744 _]
              tunnel: [w5743 _] -> w5500
              frame #0 {
                n2619 = Unbundle By Name(w5744) -> ("FRAME_TRANSFER"=w5743:bool)
              }
              frame #1 {
                # "closed"
                n2620 = Bundle By Name(cluster=w5748, "SHUTTER_MODE"=u8 2, "FRAME_TRANSFER"=FALSE) -> (w5747:T31)
              }
            }
            n2621 = call-dynamic "Read target cluster.vi"("error in (no error)"=w5540, "Channel in"=w5545) -> ("error out"=w5539:errorcluster, "target cluster"=w5541:T31, "Channel out"=w5537:refnum<class "Channel.lvclass">)  [unwired: 7 in]
            n2622 = stacked-sequence {
              tunnel: [_ w5778] -> w5543
              tunnel: w5541 -> [_ w5777]
              tunnel: w5541 -> [w5775 _]
              tunnel: [w5774 _] -> w5550
              frame #0 {
                n2623 = Unbundle By Name(w5775) -> ("FRAME_TRANSFER"=w5774:bool)
              }
              frame #1 {
                # "closed"
                n2624 = Bundle By Name(cluster=w5777, "SHUTTER_MODE"=u8 2, "FRAME_TRANSFER"=FALSE) -> (w5778:T31)
              }
            }
            n2625 = property on="Exptime ch2" class="DigNum (strict)"("Value"=w5707) -> ()  [unwired: 2 in, 2 out]
            n2626 = call-dynamic "Read target cluster.vi"("error in (no error)"=w5644, "Channel in"=w5648) -> ("error out"=w5643:errorcluster, "target cluster"=w5646:T31, "Channel out"=w5647:refnum<class "Channel.lvclass">)  [unwired: 7 in]
            n2627 = stacked-sequence {
              tunnel: [_ w5841] -> w5652
              tunnel: w5646 -> [_ w5838]
              tunnel: w5646 -> [w5837 _]
              tunnel: [w5836 _] -> w5656
              frame #0 {
                n2628 = Unbundle By Name(w5837) -> ("FRAME_TRANSFER"=w5836:bool)
              }
              frame #1 {
                # "closed"
                n2629 = Bundle By Name(cluster=w5838, "SHUTTER_MODE"=u8 2, "FRAME_TRANSFER"=FALSE) -> (w5841:T31)
              }
            }
            n2630 = call-dynamic "Write PREV_FT.vi"("error in (no error)"=w5594, "PREV_FT"=w5601, "Interface in"=w5597) -> ("error out"=w5591:errorcluster, "Interface out"=w5587:refnum<class "Interface.lvclass">)  [unwired: 7 in]
            n2631 = call-dynamic "Write PREV_FT.vi"("error in (no error)"=w5490, "PREV_FT"=w5500, "Interface in"=w5496) -> ("error out"=w5489:errorcluster, "Interface out"=w5495:refnum<class "Interface.lvclass">)  [unwired: 7 in]
